vi "Get Top Level Library Index.vi"(8 "error in":errorcluster, 11 "sourceItems":refnum<class "AB_Source.lvclass">[](array[class])) -> (0 "error out":errorcluster, 2 "Index":i32, 3 "sourceItems out":refnum<class "AB_Source.lvclass">[](array[class]))   [LabVIEW 2020, in "NI_AB_API_PPL.lvclass"]
uses:
  <vilib>/AppBuilder/AB_API/PPL/NI_AB_API_PPL.lvclass
  <vilib>/AppBuilder/AB_Classes/Source/AB_Source.lvclass
  <vilib>/AppBuilder/AB_Classes/Source/Library/AB_Source_Library.lvclass
  <vilib>/AppBuilder/AB_API/PPL/NI_AB_API_PPL.lvclass/NI_AB_API_PPL.ctl
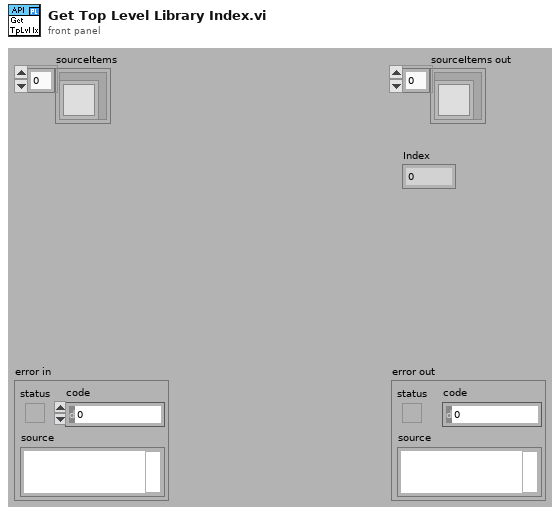
[diagram p1: front panel]
types:
  T1 = typedef "AB_Source_Library.ctl" = cluster{"relinkCallers":bool, "atomicCopy":bool, "allowMissingMembers":bool, "eng_newDelimitedName":string, "eng_hasNonVILinks":bool, "eng_reference":refnum<vi>, "LVLIBPtopLevel":bool}
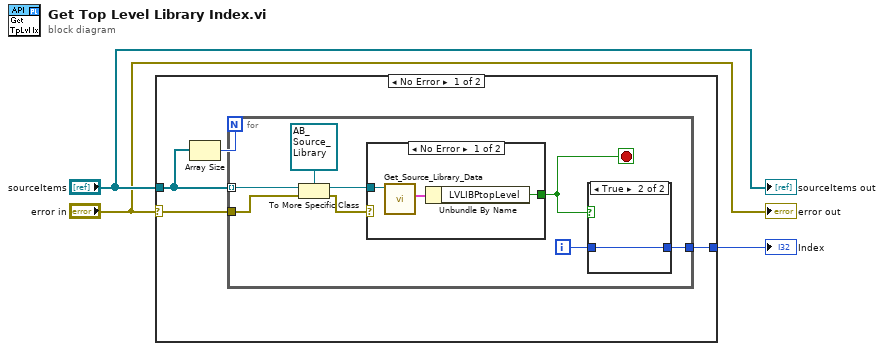
[diagram p0: block diagram]
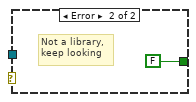
[diagram p2: hidden frame]
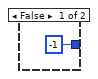
[diagram p3: hidden frame]
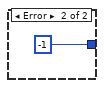
[diagram p4: hidden frame]
diagram:
  n1 = case shown="No Error" "error in" {
    selector: "error in" -> [w4 _]
    tunnel: "sourceItems" -> [w7 _]
    tunnel: [w5 -1] -> w3
    frame No Error {
      n2 = Array Size(array=w7) -> (size(s)=w6:i32)
      n3 = for {
        N: w6 -> [_]
        tunnel: w7 -> [w11] mode=indexing
        tunnel: [w14] -> w5
        tunnel: w4 -> [w10]
        i -> [w15]
        stop <- w9 stop-if-true
        n4 = To More Specific Class(target class=refnum<class "AB_Source_Library.lvclass"> refnum ("AB_Source_Library.lvclass"), reference=w11, error in=w10) -> (specific class reference=w13:refnum<class "AB_Source_Library.lvclass">, error out=w8:errorcluster)
        n5 = case shown="No Error" w8 {
          tunnel: w13 -> [w18 _]
          tunnel: [w16 FALSE ("LVLIBPtopLevel")] -> w9
          frame No Error {
            n6 = call <vilib>:"Get_Source_Library_Data.vi"("Class in"=w18) -> ("data"=w17:T1)  [unwired: 8 in, 2 out]
            n7 = Unbundle By Name(w17) -> ("LVLIBPtopLevel"=w16:bool)
          }
          frame Error {
            # "Not a library, \nkeep looking"
          }
        }
        n8 = case shown="True" w9 {
          tunnel: w15 -> [_ w21]
          tunnel: [-1 w21] -> w14
          frame False {
          }
          frame True {
          }
        }
      }
    }
    frame Error {
    }
  }
  "Index" <- w3
  "error out" <- "error in"
  "sourceItems out" <- "sourceItems"
